vi "To Euler Angles.vi"(8 "error in":errorcluster, 11 "Orient3d in":refnum<class "Orient3d.lvclass">) -> (0 "error out":errorcluster, 1 "phi/roll":dbl, 2 "theta/pitch":dbl, 3 "psi/yaw":dbl)   [LabVIEW 2024, in "Orient3d.lvclass"]
uses:
  Orient3d.lvclass
  Orient3d.lvclass/Orient3d.ctl
panel:
  # "Uses angle conventions from\nhttps://en.wikipedia.org/wiki/Conversion_between_quaternions_and_Euler_angles"
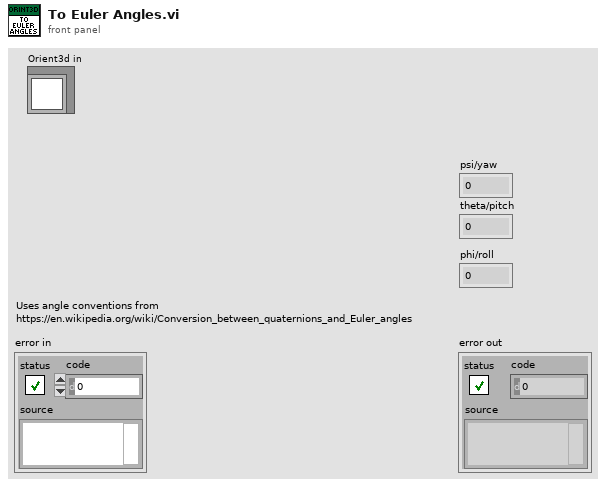
[diagram p1: front panel]
types:
  T1 = typedef "Quaternion.ctl" = cluster{"x":dbl, "y":dbl, "z":dbl, "w":dbl}
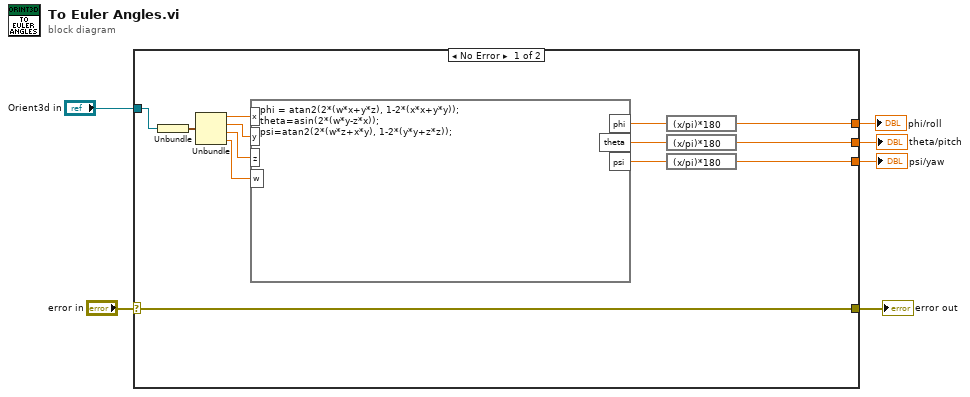
[diagram p0: block diagram]
diagram:
  n1 = case shown="No Error" "error in" {
    selector: "error in" -> [w19 w20]
    tunnel: [w19 w20] -> w5
    tunnel: "Orient3d in" -> [w18 _]
    tunnel: [w9 _] -> w3
    tunnel: [w8 _] -> w2
    tunnel: [w7 _] -> w1
    frame No Error {
      n2 = Unbundle(w18) -> (w17:T1)
      n3 = Unbundle(w17) -> ("x"=w16:dbl, "y"=w15:dbl, "z"=w14:dbl, "w"=w13:dbl)
      n4 = formula code="phi = atan2(2*(w*x+y*z), 1-2*(x*x+y*y));\ntheta=asin(2*(w*y-z*x));\npsi=atan2(2*(w*z+x*y), 1-2*(y*y+z*z));"("x"=w16, "y"=w15, "z"=w14, "w"=w13) -> ("phi"=w12:dbl, "theta"=w10:dbl, "psi"=w11:dbl)
      n5 = expression code="(x/pi)*180" ("degrees to radians")(w12) -> (w9:dbl)
      n6 = expression code="(x/pi)*180" ("degrees to radians")(w10) -> (w8:dbl)
      n7 = expression code="(x/pi)*180" ("degrees to radians")(w11) -> (w7:dbl)
    }
    frame Error {
    }
  }
  "error out" <- w5
  "psi/yaw" <- w1
  "theta/pitch" <- w2
  "phi/roll" <- w3
